vi "Angles to Targets.vi"(9 "Pixel Width":dbl format="%#_13g", 10 "Camera Type":T1=enum."MS HD3000 square", 11 "Targets In":T2(array[cluster])) -> (3 "Target Angle":dbl[](array[numeric]))   [LabVIEW 2015]
uses:
  Program Files (x86)/National Instruments/LabVIEW 2015/examples/FRC/roboRIO/Vision/2016 Vision Example/Vision Support Code/Camera Types.ctl
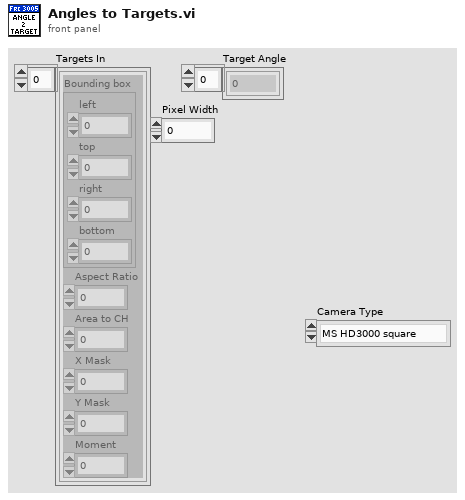
[diagram p1: front panel]
types:
  T1 = typedef "Camera Types.ctl" = enum16{"206", "1011", "1013", "MS HD3000 square", "MS HD3000 640x480"}
  T2 = cluster{"Bounding box":cluster{"left":dbl, "top":dbl, "right":dbl, "bottom":dbl}, "Aspect Ratio":dbl, "Area to CH":dbl, "X Mask":dbl, "Y Mask":dbl, "Moment":dbl}[]
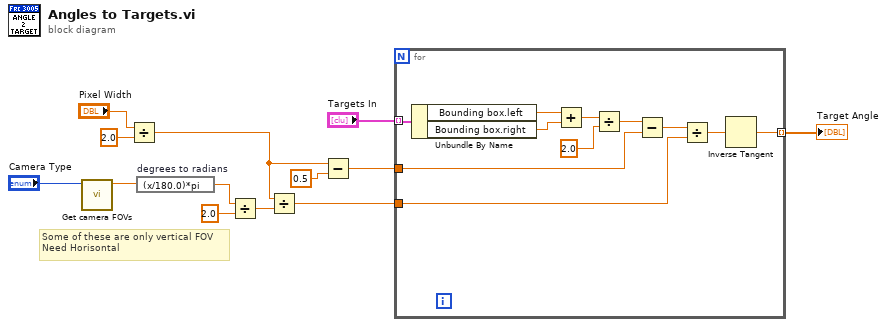
[diagram p0: block diagram]
diagram:
  # "Some of these are only vertical FOV\nNeed Horisontal"
  n1 = call "Get camera FOVs.vi"("Camera Type"="Camera Type") -> ("FOV"=w10:dbl)  [unwired: 9 in, 1 out]
  n2 = Divide(x="Pixel Width", y=2.0) -> (x/y=w4:dbl)
  n3 = expression code="(x/180.0)*pi" "degrees to radians"(w10) -> (w9:dbl)
  n4 = Divide(x=w9, y=2.0) -> (x/y=w6:dbl)
  n5 = Divide(x=w4, y=w6) -> (x/y=w5:dbl)
  n6 = Subtract(x=w4, y=0.5) -> (x-y=w2:dbl)
  n7 = for {
    tunnel: "Targets In" -> [w22] mode=indexing
    tunnel: w5 -> [w16]
    tunnel: w2 -> [w19]
    tunnel: [w14] -> w1 mode=indexing
    n8 = Unbundle By Name(w22) -> ("Bounding box.left"=w21:dbl, "Bounding box.right"=w20:dbl)
    n9 = Add(x=w21, y=w20) -> (x+y=w23:dbl)
    n10 = Divide(x=w23, y=2.0) -> (x/y=w18:dbl)
    n11 = Subtract(x=w18, y=w19) -> (x-y=w17:dbl)
    n12 = Divide(x=w17, y=w16) -> (x/y=w15:dbl)
    n13 = Inverse Tangent(1:w15) -> (0:w14:dbl)
  }
  "Target Angle" <- w1
